vi "xy_graph.vi"() -> ()   [LabVIEW 2021]
panel:
  in  "x":ext
  in  "a":dbl
  in  "v0":dbl
  out "XY Graph":cluster{dbl[], dbl[]}(graph)
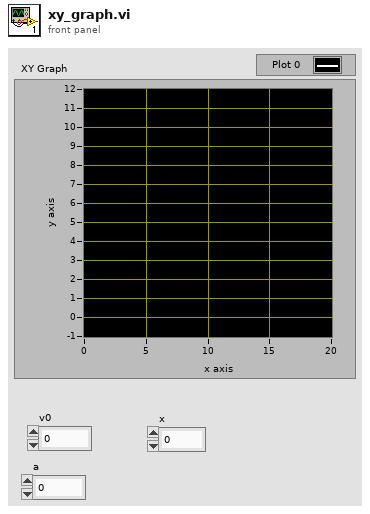
[diagram p1: front panel]
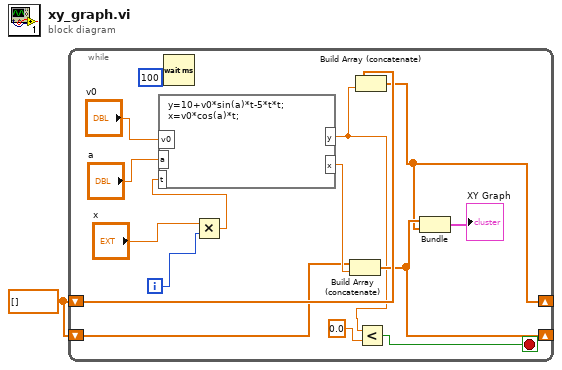
[diagram p0: block diagram]
diagram:
  w1 = dbl[] []
  n1 = while {
    shift-right: [w6] -> _
    shift-left: w1 -> [w10]
    shift-right: [w5] -> _
    shift-left: w1 -> [w11]
    i -> [w15]
    stop <- w2 stop-if-true
    n2 = Wait (ms)(milliseconds to wait=u32 100) -> ()  [unwired: 1 out]
    n3 = Multiply(x="x", y=w15) -> (x*y=w14:ext)
    n4 = formula code="y=10+v0*sin(a)*t-5*t*t;\nx=v0*cos(a)*t;"("v0"="v0", "a"="a", "t"=w14) -> ("x"=w12:dbl, "y"=w4:dbl)
    n5 = Build Array (concatenate)(w10, w12) -> (w6:dbl[])
    n6 = Build Array (concatenate)(w11, w4) -> (w5:dbl[])
    n7 = Less?(x=w4, y=0.0) -> (x < y?=w2:bool)
    n8 = Bundle(w6, w5) -> (→"XY Graph":cluster{dbl[], dbl[]})  [unwired: 1 in]
  }
